vi "Stop Core.vi"(10 "final error code":i32, 11 "PredictiveMaintenance in":refnum<class "PredictiveMaintenance.lvclass">) -> (3 "PredictiveMaintenance out":refnum<class "PredictiveMaintenance.lvclass">)   [LabVIEW 2019, in "PredictiveMaintenance.lvlib" / "PredictiveMaintenance.lvclass"]
doc: "(<B>Filename</B>: Actor Framework.lvlib:Actor.lvclass:Stop Core.vi)\n\nDefines what the actor does before it stops. Use the <B>final error code</B> input to determine whether the actor shut down in response to an error.\n\nBy default, this method passes the Stop message along to all auto-stop nested actors. A descendant class may override this method to define additional behavior, such as shutting down any processes the actor initiated in its override of the Actor Core method."
uses:
  PredictiveMaintenance.lvclass
  PredictiveMaintenance.lvclass/PredictiveMaintenance.ctl
  <vilib>/ActorFramework/Actor/Actor.lvclass
  ConfigClass/ConfigClass/ConfigClass.lvclass
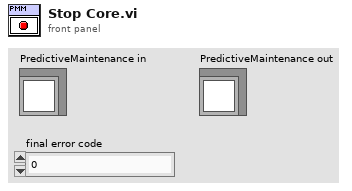
[diagram p1: front panel]
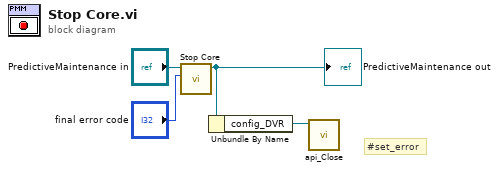
[diagram p0: block diagram]
diagram:
  # "#set_error"
  n1 = call-parent "Stop Core.vi"("final error code"="final error code", "Actor in"="PredictiveMaintenance in") -> ("Actor out"=w2:refnum<class "PredictiveMaintenance.lvclass">)  [unwired: 9 in]
  "PredictiveMaintenance out" <- w2
  n2 = Unbundle By Name(w2) -> ("config_DVR"=w1:refnum<data-value>)
  n3 = call "api_Close.vi"("ConfigClass_DVR"=w1) -> ()  [unwired: 9 in, 2 out]
